vi "L0_Baseline_File_Create.vi"(1 "input cluster":T1, 2 "Serial Number":string="testFile") -> (0 "appended path":path)   [LabVIEW 2012]
uses:
  <vilib>/Utility/NIReport.llb/NI_report.lvclass
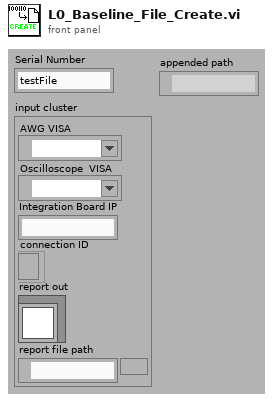
[diagram p1: front panel]
types:
  T1 = cluster{"AWG VISA":refnum<visa-resource-name>, "Oscilloscope  VISA ":refnum<visa-resource-name>, "Integration Board IP":string, "connection ID":refnum<k5>, "report out":refnum<class "NI_report.lvclass">, "report file path":path}
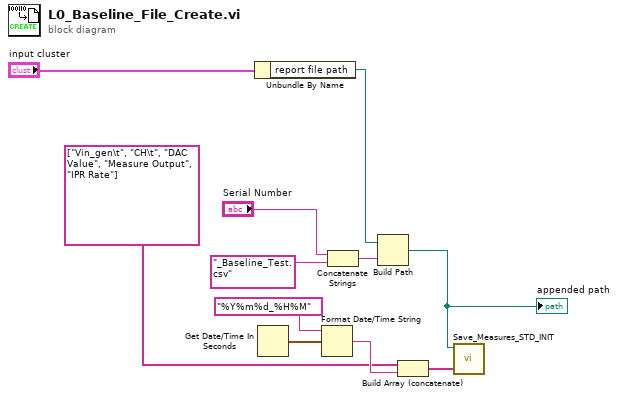
[diagram p0: block diagram]
diagram:
  n1 = Unbundle By Name("input cluster") -> ("report file path"=w5:path)
  n2 = Get Date/Time In Seconds() -> (seconds since 1Jan1904=w10:timestamp)
  n3 = Format Date/Time String(time format string (%c)="%Y%m%d_%H%M", seconds (now)=w10) -> (date/time string=w8:string)  [unwired: 1 in]
  n4 = Concatenate Strings("Serial Number", "_Baseline_Test.csv" ("format string")) -> (w6:string)
  n5 = Build Path(base path=w5, name or relative path=w6) -> (appended path=w3:path)
  "appended path" <- w3
  n6 = Build Array (concatenate)(string[] ["Vin_gen\t", "CH\t", "DAC Value", "Measure Output", "IPR Rate"] ("appended array"), w8) -> (w11:string[])
  n7 = call "Save_Measures_STD_INIT.vi"("appended array"=w11, "file path (dialog if empty)"=w3) -> ()  [unwired: 10 in]
